vi "Compute Target Distances and Angles.vi"(9 "Camera Type":enum16{"206", "1011", "1013"}(ring), 10 "Target Info":T4(array[cluster]), 11 "Image in":T3) -> (0 "Distances":T2(array[cluster]), 2 "Target Info":T5(array[cluster]), 3 "Image out":T3)   [LabVIEW 2013]
uses:
  TargetType.ctl
  <vilib>/vision/Image Controls.llb/IMAQ Image.ctl
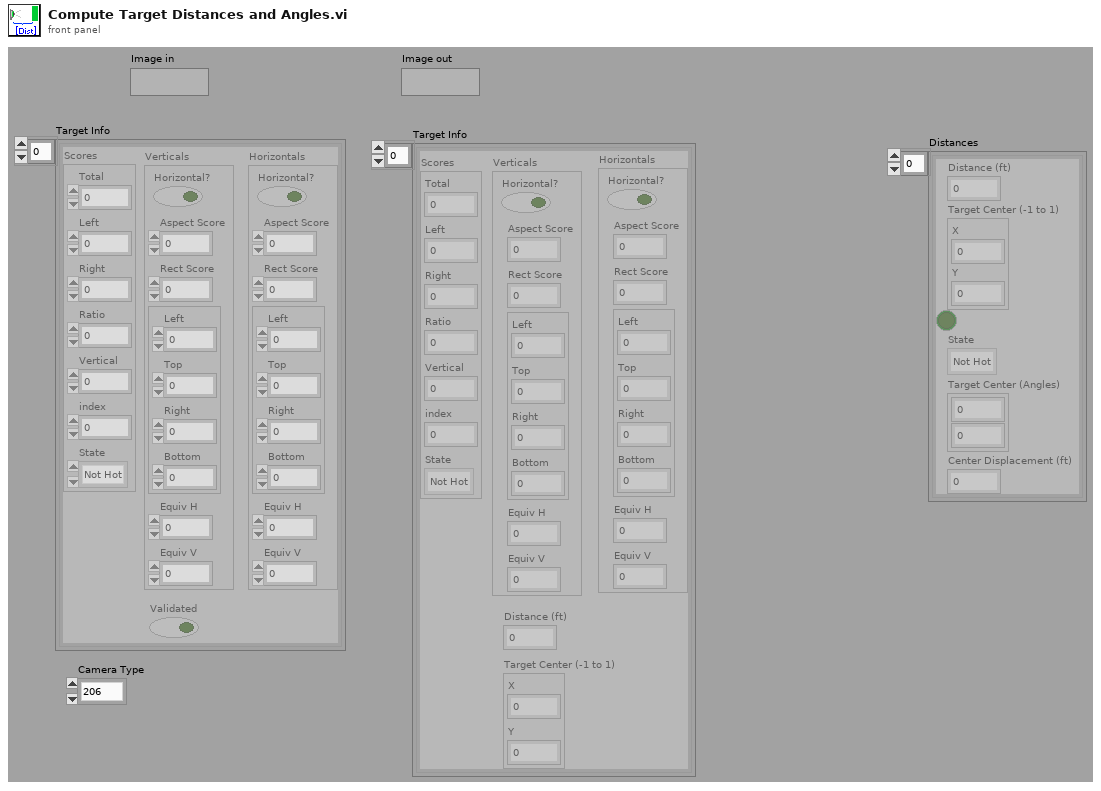
[diagram p1: front panel]
types:
  T1 = typedef "TargetType.ctl" = enum16{"Not Hot", "Hot"}
  T2 = cluster{"Distance (ft)":dbl, "Target Center (-1 to 1)":cluster{"X":dbl, "Y":dbl}, bool, "State":T1, "Target Center (Angles)":cluster{dbl, dbl}, "Center Displacement (ft)":dbl}[]
  T3 = typedef "IMAQ Image.ctl" = refnum<image>
  T4 = cluster{"Scores":cluster{"Total":dbl, "Left":dbl, "Right":dbl, "Ratio":dbl, "Vertical":dbl, "index":i32, "State":T1}, "Verticals":cluster{"Horizontal?":bool, "Aspect Score":dbl, "Rect Score":dbl, cluster{"Left":dbl, "Top":dbl, "Right":dbl, "Bottom":dbl}, "Equiv H":dbl, "Equiv V":dbl}, "Horizontals":cluster{"Horizontal?":bool, "Aspect Score":dbl, "Rect Score":dbl, cluster{"Left":dbl, "Top":dbl, "Right":dbl, "Bottom":dbl}, "Equiv H":dbl, "Equiv V":dbl}, "Validated":bool}[]
  T5 = cluster{"Scores":cluster{"Total":dbl, "Left":dbl, "Right":dbl, "Ratio":dbl, "Vertical":dbl, "index":i32, "State":T1}, "Verticals":cluster{"Horizontal?":bool, "Aspect Score":dbl, "Rect Score":dbl, cluster{"Left":dbl, "Top":dbl, "Right":dbl, "Bottom":dbl}, "Equiv H":dbl, "Equiv V":dbl}, "Horizontals":cluster{"Horizontal?":bool, "Aspect Score":dbl, "Rect Score":dbl, cluster{"Left":dbl, "Top":dbl, "Right":dbl, "Bottom":dbl}, "Equiv H":dbl, "Equiv V":dbl}, "Distance (ft)":dbl, "Target Center (-1 to 1)":cluster{"X":dbl, "Y":dbl}}[]
  T6 = cluster{"Total":dbl, "Left":dbl, "Right":dbl, "Ratio":dbl, "Vertical":dbl, "index":i32, "State":T1}
  T7 = cluster{"Horizontal?":bool, "Aspect Score":dbl, "Rect Score":dbl, cluster{"Left":dbl, "Top":dbl, "Right":dbl, "Bottom":dbl}, "Equiv H":dbl, "Equiv V":dbl}
  T8 = cluster{"Scores":cluster{"Total":dbl, "Left":dbl, "Right":dbl, "Ratio":dbl, "Vertical":dbl, "index":i32, "State":T1}, "Verticals":cluster{"Horizontal?":bool, "Aspect Score":dbl, "Rect Score":dbl, cluster{"Left":dbl, "Top":dbl, "Right":dbl, "Bottom":dbl}, "Equiv H":dbl, "Equiv V":dbl}, "Horizontals":cluster{"Horizontal?":bool, "Aspect Score":dbl, "Rect Score":dbl, cluster{"Left":dbl, "Top":dbl, "Right":dbl, "Bottom":dbl}, "Equiv H":dbl, "Equiv V":dbl}, "Distance (ft)":dbl, "Target Center (-1 to 1)":cluster{"X":dbl, "Y":dbl}}
  T9 = cluster{"Distance (ft)":dbl, "Target Center (-1 to 1)":cluster{"X":dbl, "Y":dbl}, bool, "State":T1, "Target Center (Angles)":cluster{dbl, dbl}, "Center Displacement (ft)":dbl}
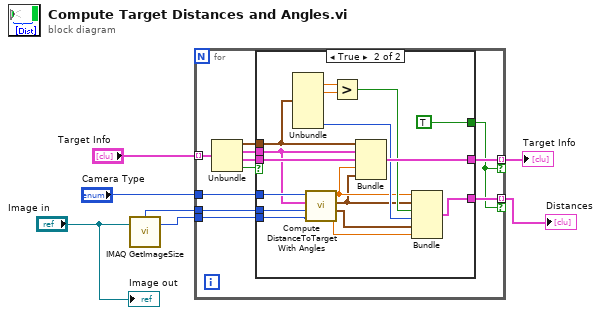
[diagram p0: block diagram]
diagram:
  n1 = call "IMAQ GetImageSize"("Image"="Image in") -> ("Y Resolution"=w6:i32, "X Resolution"=w5:i32)  [unwired: 3 in, 1 out]
  n2 = for {
    tunnel: "Target Info" -> [w18] mode=indexing
    tunnel: "Camera Type" -> [w15]
    tunnel: w5 -> [w14]
    tunnel: w6 -> [w13]
    tunnel: [w10] -> w7 mode=indexing if=w8
    tunnel: [w9] -> w1 mode=indexing if=w8
    n3 = Unbundle(w18) -> ("Scores"=w12:T6, "Verticals"=w16:T7, "Horizontals"=w11:T7, "Validated"=w17:bool)
    n4 = case shown="True" w17 {
      tunnel: w16 -> [_ w25]
      tunnel: w15 -> [_ w26]
      tunnel: w14 -> [_ w24]
      tunnel: w13 -> [_ w23]
      tunnel: w12 -> [_ w31]
      tunnel: w11 -> [_ w35]
      tunnel: [_ w34] -> w10
      tunnel: [_ TRUE] -> w8
      tunnel: [_ w32] -> w9
      frame False {
      }
      frame True {
        n5 = Unbundle(w31) -> ("Left"=w30:dbl, "Right"=w29:dbl, "State"=w27:T1)  [unwired: 4 out]
        n6 = call "Compute DistanceToTarget With Angles.vi"("Y Image Resolution"=w23, "X Image Resolution"=w24, "Vertical Strip"=w25, "Camera Type"=w26) -> ("Center Displacement (ft)"=w19:dbl, "Target Center (Angles)"=w20:cluster{dbl, dbl}, "Target Center (-1 to 1)"=w21:cluster{"X":dbl, "Y":dbl}, "Distance (ft)"=w22:dbl)  [unwired: 4 in]
        n7 = Greater?(x=w30, y=w29) -> (0:w28:bool)
        n8 = Bundle("Scores"=w31, "Verticals"=w25, "Horizontals"=w35, "Distance (ft)"=w22, "Target Center (-1 to 1)"=w21) -> (w34:T8)  [unwired: 1 in]
        n9 = Bundle("Distance (ft)"=w22, "Target Center (-1 to 1)"=w21, w28, "State"=w27, "Target Center (Angles)"=w20, "Center Displacement (ft)"=w19) -> (w32:T9)  [unwired: 1 in]
      }
    }
  }
  "Target Info" <- w7
  "Distances" <- w1
  "Image out" <- "Image in"
